vi "from string.vi"(8 "error in":errorcluster, 9 "data":string, 10 "version":string, 11 "tag bus configurable plugin module configuration in":refnum<class "tag bus processing plugin module configuration.lvclass">) -> (0 "error out":errorcluster, 3 "tag bus configurable plugin module configuration out":refnum<class "tag bus processing plugin module configuration.lvclass">)   [LabVIEW 2013, in "tag bus processing plugin module configuration.lvclass"]
doc: "Provides an interface for loading a module configuration from a file or other serialized data source. It is recommended that all children of this class store data in two sets--data required for its own initialization, and any data required for parent initialization--and that each implementation uses the <b>Call Parent Method</b> primitive to de-serialize parent information. As a result, it is expected that every module configuration class calls <b>component configuration.lvclass:From String.vi</b>."
uses:
  tag bus processing plugin module configuration.lvclass
  <vilib>/NI/Tag Bus Module Framework/module configuration/TBM module configuration.lvclass
  <vilib>/NI/Tag Bus Module Framework/channel/TBM channel.lvclass
  processing channels.ctl
  <vilib>/NI/Configuration Framework/serializable configuration/NISE_CEF_serializable configuration.lvclass
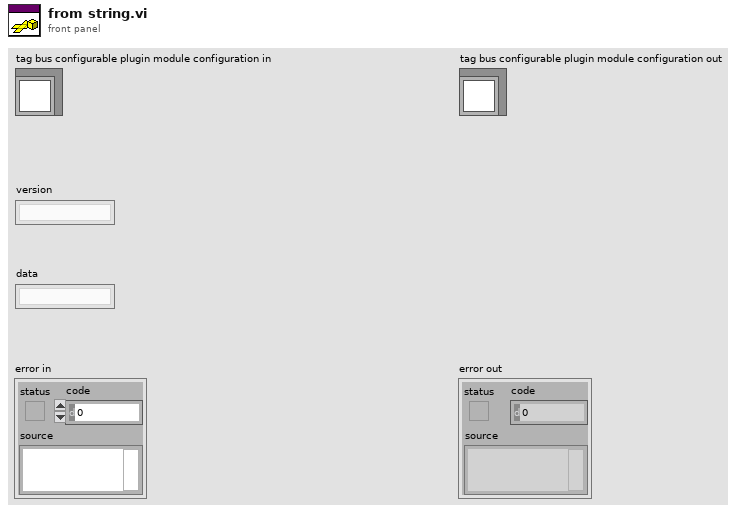
[diagram p1: front panel]
types:
  T1 = typedef "tag bus processing plugin module configuration.lvclass/processing channels.ctl" = cluster{"parameter":refnum<class "TBM channel.lvclass">, "result":refnum<class "TBM channel.lvclass">}
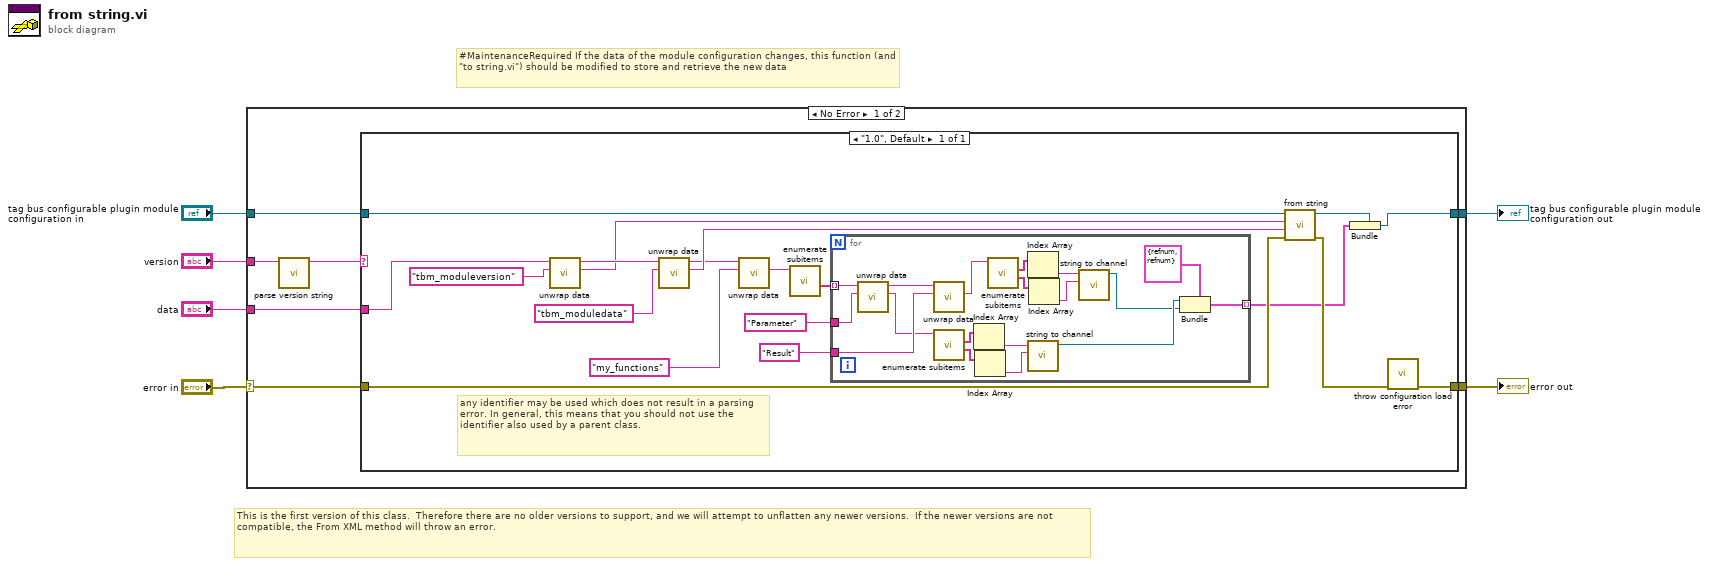
[diagram p0: block diagram]
diagram:
  # "#MaintenanceRequired If the data of the module configuration changes, this function (and \"to string.vi\") should be modified to store and retrieve the new data"
  # "This is the first version of this class.  Therefore there are no older versions to support, and we will attempt to unflatten any newer versions.  If the newer versions are not compatible, the From XML method will throw an error."
  n1 = case shown="No Error" "error in" {
    selector: "error in" -> [w7 w52]
    tunnel: "data" -> [w13 _]
    tunnel: "tag bus configurable plugin module configuration in" -> [w12 w51]
    tunnel: [w11 w51] -> w2
    tunnel: [w10 w52] -> w1
    tunnel: "version" -> [w9 _]
    frame No Error {
      n2 = call <vilib>:"parse version string.vi"("full version"=w9) -> ("major.minor version"=w8:string)  [unwired: 7 in, 3 out]
      n3 = case shown="\"1.0\", Default" w8 {
        tunnel: w13 -> [w28]
        tunnel: w7 -> [w27]
        tunnel: w12 -> [w32]
        tunnel: [w22] -> w11
        tunnel: [w30] -> w10
        frame "1.0", Default {
          # "any identifier may be used which does not result in a parsing error. In general, this means that you should not use the identifier also used by a parent class."
          n4 = call <vilib>:"unwrap data.vi"("identifier"="tbm_moduleversion" ("additional identifier"), "data to unwrap"=w28) -> ("unwrapped data"=w23:string, "remaining string"=w29:string)  [unwired: 8 in]
          n5 = call <vilib>:"unwrap data.vi"("identifier"="tbm_moduledata" ("additional identifier"), "data to unwrap"=w29) -> ("unwrapped data"=w25:string, "remaining string"=w21:string)  [unwired: 8 in]
          n6 = call <vilib>:"unwrap data.vi"("identifier"="my_functions" ("additional identifier"), "data to unwrap"=w21) -> ("unwrapped data"=w18:string)  [unwired: 8 in, 1 out]
          n7 = call <vilib>:"enumerate subitems.vi"("data to enumerate"=w18) -> ("associated data"=w17:string[])  [unwired: 8 in, 2 out]
          n8 = for {
            tunnel: w17 -> [w50] mode=indexing
            tunnel: "Parameter" ("identifier") -> [w49]
            tunnel: "Result" ("identifier") -> [w47]
            tunnel: [w33] -> w14 mode=indexing
            n9 = call <vilib>:"unwrap data.vi"("identifier"=w49, "data to unwrap"=w50) -> ("unwrapped data"=w46:string, "remaining string"=w48:string)  [unwired: 8 in]
            n10 = call <vilib>:"unwrap data.vi"("identifier"=w47, "data to unwrap"=w48) -> ("unwrapped data"=w41:string)  [unwired: 8 in, 1 out]
            n11 = call <vilib>:"enumerate subitems.vi"("data to enumerate"=w46) -> ("associated data"=w44:string[], "discovered subitems"=w45:string[])  [unwired: 8 in, 1 out]
            n12 = Index Array(array=w45) -> (element=w40:string)  [unwired: 1 in]
            n13 = Index Array(array=w44) -> (element=w39:string)  [unwired: 1 in]
            n14 = call <vilib>:"enumerate subitems.vi"("data to enumerate"=w41) -> ("associated data"=w43:string[], "discovered subitems"=w42:string[])  [unwired: 8 in, 1 out]
            n15 = Index Array(array=w42) -> (element=w37:string)  [unwired: 1 in]
            n16 = call <vilib>:"string to channel.vi"("channel data"=w39, "identifier"=w40) -> ("channel in"=w35:refnum<class "TBM channel.lvclass">)  [unwired: 9 in]
            n17 = Index Array(array=w43) -> (element=w38:string)  [unwired: 1 in]
            n18 = call <vilib>:"string to channel.vi"("channel data"=w38, "identifier"=w37) -> ("channel in"=w34:refnum<class "TBM channel.lvclass">)  [unwired: 9 in]
            n19 = Bundle(cluster=T1 {"parameter"=refnum, "result"=refnum} ("processing cluster"), "parameter"=w35, "result"=w34) -> (w33:T1)
          }
          n20 = call-parent "from string.vi"("error in"=w27, "data"=w25, "version"=w23, "module configuration in"=w32) -> ("error out"=w19:errorcluster, "module configuration out"=w31:refnum<class "tag bus processing plugin module configuration.lvclass">)  [unwired: 6 in]
          n21 = Bundle(cluster=w31, w14) -> (w22:refnum<class "tag bus processing plugin module configuration.lvclass">)
          n22 = call <vilib>:"throw configuration load error.vi"("error in"=w19) -> ("error out"=w30:errorcluster)  [unwired: 10 in]
        }
      }
    }
    frame Error {
    }
  }
  "error out" <- w1
  "tag bus configurable plugin module configuration out" <- w2
